vi "SysDef.Property.Set.DependentFile.vi"(8 "error in (no error)":errorcluster, 9 "Value":T1, 10 "Property Name":string, 11 "nodeID":u64) -> (0 "error out":errorcluster, 3 "nodeID out":u64)   [LabVIEW 2015, in "Import - Export CD Config Utility.lvlib"]
uses:
  Import - Export CD Config Utility.lvlib
  _Types/Property.DependentFile.ctl
  <vilib>/NI Veristand/Custom Device API/Dependent File Optional Info.ctl
  <vilib>/NI Veristand/Custom Device API/Set Item Property (Dependent File).vi
  NationalInstruments.VeriStand.SystemDefinitionAPI
  <vilib>/NI Veristand/Custom Device API/Custom Device API.lvlib
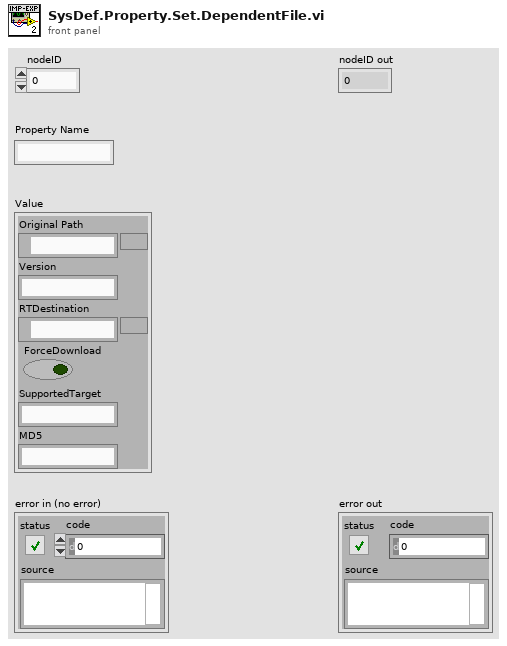
[diagram p1: front panel]
types:
  T1 = typedef "Import - Export CD Config Utility.lvlib/Property.DependentFile.ctl" = cluster{"Original Path":path, "Version":string, "RTDestination":path, "ForceDownload":bool, "SupportedTarget":string, "MD5":string}
  T2 = typedef "Custom Device API.lvlib/Dependent File Optional Info.ctl" = cluster{"Version":string, "RTDestination":path, "ForceDownload":bool, "SupportedTarget":string, "MD5":string}
  T3 = typedef "Custom Device API.lvlib/Custom Device Item Ref.ctl" = u64
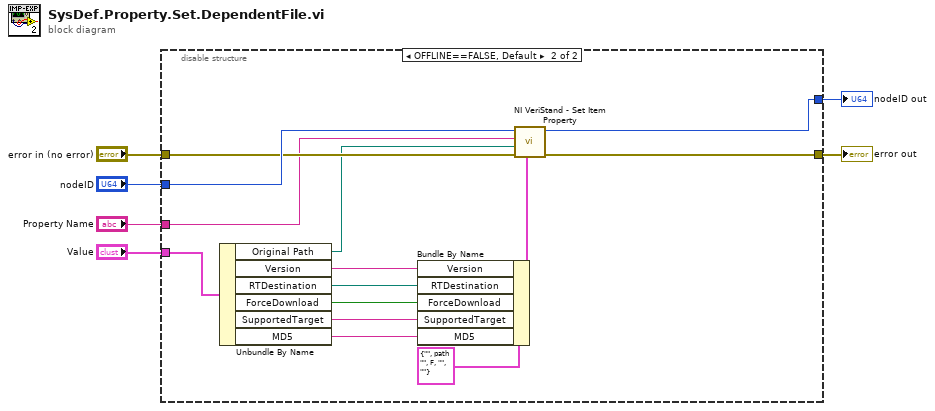
[diagram p0: block diagram]
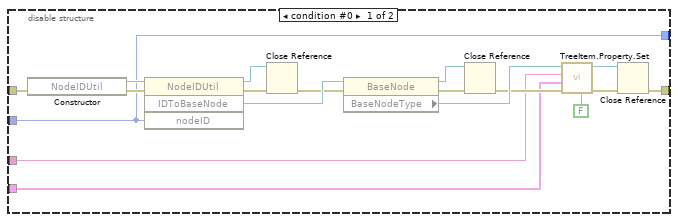
[diagram p2: hidden frame]
diagram:
  n1 = disable-structure shown="OFFLINE==FALSE, Default" {
    disable-tunnel: "error in (no error)" -> [w17 w37]
    disable-tunnel: "nodeID" -> [w7 w38]
    disable-tunnel: [w11 w35] -> w4
    disable-tunnel: "Property Name" -> [w10 w36]
    disable-tunnel: "Value" -> [w9 w33]
    disable-tunnel: [w7 w34] -> w1
    frame condition #0 {
      n2 = constructor class="NodeIDUtil"(error in=w17) -> (reference out=w24:refnum<k24>, error out=w23:errorcluster)  [unwired: 2 in, 1 out]
      n3 = invoke class="NodeIDUtil" method="IDToBaseNode"(reference=w24, error in=w23, "nodeID"=w7) -> (reference out=w18:refnum<k24>, error out=w20:errorcluster, "IDToBaseNode"=w22:refnum<k24>)  [unwired: 1 in, 1 out]
      n4 = Close Reference(reference=w18, error in (no error)=w20) -> (error out=w19:errorcluster)
      n5 = property class="BaseNode"(reference=w22, error in=w19) -> (reference out=w16:refnum<k24>, error out=w15:errorcluster, "BaseNodeType"=w21:refnum<k24>)
      n6 = Close Reference(reference=w16, error in (no error)=w15) -> (error out=w14:errorcluster)
      n7 = call "TreeItem.Property.Set.vi"("Set String as Binary"=FALSE, "error in (no error)"=w14, "Value"=w9, "Property Name"=w10, "BaseNodeType"=w21) -> ("error out"=w13:errorcluster, "BaseNodeType"=w12:refnum<k24>)  [unwired: 4 in, 1 out]
      n8 = Close Reference(reference=w12, error in (no error)=w13) -> (error out=w11:errorcluster)
    }
    frame condition #1 (active) {
      n9 = Unbundle By Name(w33) -> ("Original Path"=w32:path, "Version"=w29:string, "RTDestination"=w25:path, "ForceDownload"=w26:bool, "SupportedTarget"=w27:string, "MD5"=w28:string)
      n10 = Bundle By Name(cluster=T2 {"Version"="", "RTDestination"=path "", "ForceDownload"=FALSE, "SupportedTarget"="", "MD5"=""} ("OptionalInfo"), "Version"=w29, "RTDestination"=w25, "ForceDownload"=w26, "SupportedTarget"=w27, "MD5"=w28) -> (w30:T2)
      n11 = call-poly <vilib>:"NI VeriStand - Set Item Property.vi"("OptionalInfo"=w30, "error in (no error)"=w37, "Path"=w32, "Property Name"=w36, "Item Ref in"=w38) -> ("error out"=w35:errorcluster, "Item Ref out"=w34:T3)  [unwired: 4 in, 1 out]
    }
  }
  "nodeID out" <- w1
  "error out" <- w4
